vi "SetParam.vi"(8 "error in (no error)":errorcluster caption="entrée d'erreur (pas d'erreur)", 10 "TimeSeriesSplit":cluster{"n_splits":i32, "max_train_size":string}={"n_splits"=5, "max_train_size"="None"}, 11 "TimeSeriesSplit.lvclass":refnum<class "TimeSeriesSplit.lvclass">) -> (0 "error out":errorcluster caption="sortie d'erreur", 3 "TimeSeriesSplit.lvclass":refnum<class "TimeSeriesSplit.lvclass">)   [LabVIEW 2020, in "TimeSeriesSplit.lvclass"]
doc: "Set Parameters"
uses:
  TimeSeriesSplit.lvclass
  TimeSeriesSplit.lvclass/TimeSeriesSplit.ctl
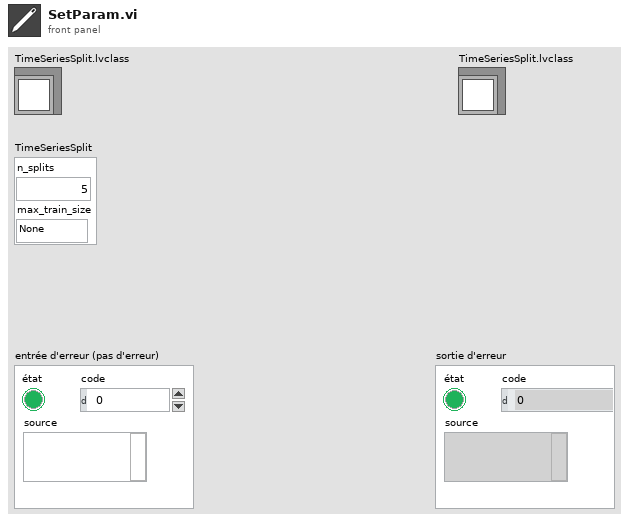
[diagram p1: front panel]
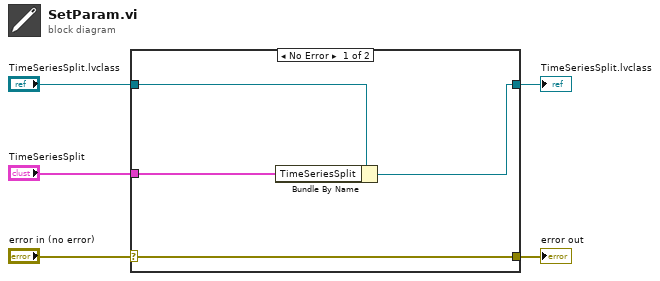
[diagram p0: block diagram]
diagram:
  n1 = case shown="No Error" "error in (no error)" {
    selector: "error in (no error)" -> [w9 w10]
    tunnel: [w9 w10] -> w4
    tunnel: [w7 w11] -> w2
    tunnel: "TimeSeriesSplit.lvclass" -> [w8 w11]
    tunnel: "TimeSeriesSplit" -> [w6 _]
    frame No Error {
      n2 = Bundle By Name(cluster=w8, "TimeSeriesSplit"=w6) -> (w7:refnum<class "TimeSeriesSplit.lvclass">)
    }
    frame Error {
    }
  }
  "error out" <- w4
  "TimeSeriesSplit.lvclass" <- w2
